vi "AskNodeForServiceProviders.vi"(0 "Service ROS":T5={"topic port"=0, "Node"="", "topic"="", "type"="", "node port"=0, "error "={"status"=FALSE, "code"=0, "source"=""}, "Direction"=enum."Node", "APIs"=[], "Update (ms)"=1, "write queue"=1}) -> (1 "Connections":T2(array[cluster]), 2 "MyState":T4, 3 "Log":T1)   [LabVIEW 2012]
uses:
  <userlib>/ROSforLV/ROS/Code/SubVIs/_ROSControl.ctl
  <userlib>/ROSforLV/ROS/Code/SubVIs/_ROSDirection.ctl
  <userlib>/ROSforLV/ROS/Code/Console/Servers/ServerSubs/MyState.ctl
  <userlib>/ROSforLV/ROS/Code/Console/Servers/ServerSubs/ROSLog.ctl
  <userlib>/ROSforLV/ROS/Code/_ROSDefinition.vi
panel:
  out "Reply":T3(array[cluster])
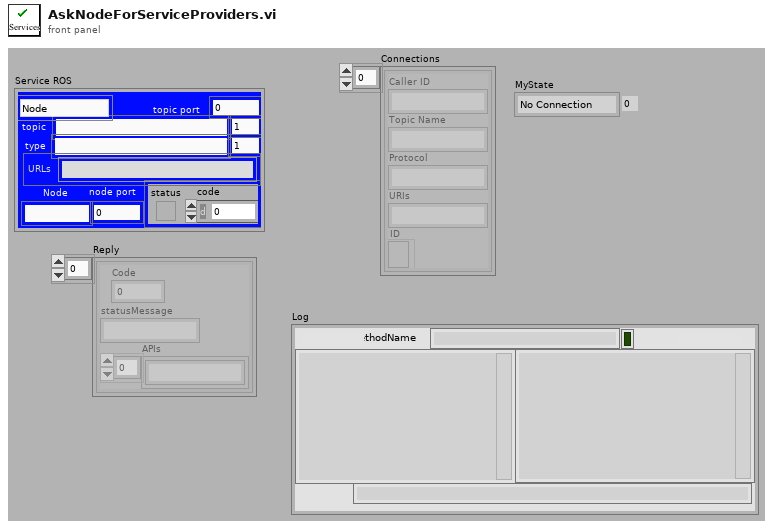
[diagram p1: front panel]
types:
  T1 = typedef "ROSLog.ctl" = cluster{"Sent":string, "Reply":string, "MethodName":string, "success":bool, "Dir1":string, "Dir2":string, "Time Stamp":string, "error":errorcluster, "Preamble":string}
  T2 = cluster{"Caller ID":string, "Topic Name":string, "Protocol":string, "URIs":string, "ID":refnum<k5>}[]
  T3 = cluster{"Code":i8, "statusMessage":string, "APIs":string[]}[]
  T4 = typedef "MyState.ctl" = enum16{"No Connection", "Registered", "Connected", "Close"}
  T5 = typedef "_ROSControl.ctl" = cluster{"topic port":u16, "Node":string, "topic":string, "type":string, "node port":u32, "error ":errorcluster, "Direction":T6, "APIs":string[], "Update (ms)":u16, "write queue":u16}
  T6 = typedef "_ROSDirection.ctl" = enum16{"Node", "Publisher", "Subscriber", "Service Client"}
  T7 = cluster{"Caller ID":string, "Topic Name":string, "Protocol":string, "URIs":string, "ID":refnum<k5>}
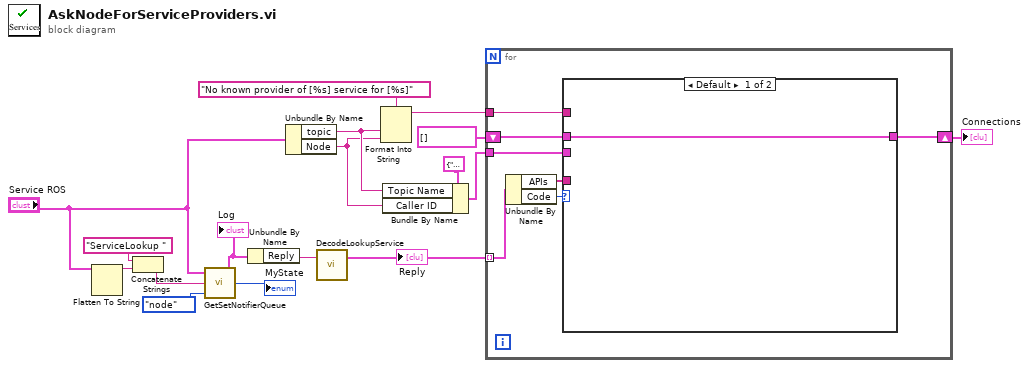
[diagram p0: block diagram]
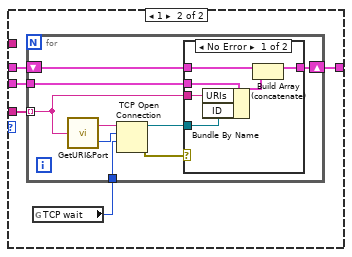
[diagram p2: hidden frame]
diagram:
  n1 = Flatten To String(anything="Service ROS") -> (data string=w15:string)  [unwired: 3 in, 2 out]
  n2 = Concatenate Strings("ServiceLookup " ("element"), w15) -> (w14:string)
  n3 = call <userlib>:"GetSetNotifierQueue.vi"("Name"=enum16{"topic", "node"}."node", "Command"=w14, "ROS"="Service ROS") -> ("MyState"=→"MyState":T4, "Log"=w12:T1)  [unwired: 1 in]
  "Log" <- w12
  n4 = Unbundle By Name(w12) -> ("Reply"=w11:string)
  n5 = Unbundle By Name("Service ROS") -> ("topic"=w8:string, "Node"=w7:string)
  n6 = call <userlib>:"DecodeLookupService.vi"("Response"=w11) -> ("Reply"=w3:T3)  [unwired: 1 in, 1 out]
  "Reply" <- w3
  n7 = Format Into String(format string="No known provider of [%s] service for [%s]", w8, w7) -> (resulting string=w4:string)  [unwired: 2 in, 1 out]
  n8 = Bundle By Name(cluster=T7 {"Caller ID"="", "Topic Name"="", "Protocol"="???", "URIs"="", "ID"=refnum} ("Subscriber"), "Topic Name"=w8, "Caller ID"=w7) -> (w6:T7)
  n9 = for {
    tunnel: w3 -> [w24] mode=indexing
    tunnel: w6 -> [w22]
    shift-right: [w20] -> w2
    shift-left: T2 [] -> [w21]
    tunnel: w4 -> [w18]
    n10 = Unbundle By Name(w24) -> ("APIs"=w23:string[], "Code"=w19:i8)
    n11 = case shown="Default" w19 {
      tunnel: w23 -> [_ w30]
      tunnel: w22 -> [_ w29]
      tunnel: w21 -> [w25 w28]
      tunnel: [w25 w27] -> w20
      tunnel: w18 -> [_ _]
      frame Default {
      }
      frame 1 {
        n12 = global read "_ROSDefinition.vi" "TCP wait"() -> (w26:i32)
        n13 = for {
          tunnel: w30 -> [w32] mode=indexing
          tunnel: w29 -> [w33]
          shift-right: [w36] -> w27
          shift-left: w28 -> [w35]
          tunnel: w26 -> [w31]
          n14 = call <userlib>:"GetURI&Port.vi"("URI in"=w32) -> ("Port"=w39:u16, "URI"=w38:string)
          n15 = TCP Open Connection(address=w38, remote port or service name=w39, timeout ms (60000)=w31) -> (connection ID=w34:refnum<k5>, error out=w37:errorcluster)  [unwired: 2 in]
          n16 = case shown="No Error" w37 {
            tunnel: [w45 w46] -> w36
            tunnel: w35 -> [w44 w46]
            tunnel: w34 -> [w41 _]
            tunnel: w33 -> [w43 _]
            tunnel: w32 -> [w42 _]
            frame No Error {
              n17 = Bundle By Name(cluster=w43, "URIs"=w42, "ID"=w41) -> (w40:T7)
              n18 = Build Array (concatenate)(w44, w40) -> (w45:T2)
            }
            frame Error {
            }
          }
        }
      }
    }
  }
  "Connections" <- w2
